vi "Motor Controller Mech Config.vi"(0 "COM port":refnum<visa-resource-name>, 5 "RS-485 addr.":u8, 7 "Encoder counting edges":u8=4, 9 "Encoder PPR":u16=256, 11 "Final drive ratio (X:1)":sgl=1.0, 12 "Close port after action":bool) -> (4 "COM port out":refnum<visa-resource-name>, 15 "Error out":errorcluster)   [LabVIEW 2020]
uses:
  ctls/CTRL_Cmd.ctl
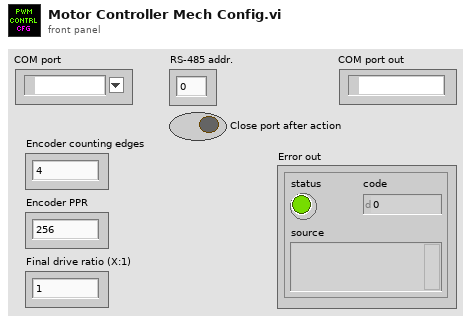
[diagram p1: front panel]
types:
  T1 = typedef "CTRL_Cmd.ctl" = string
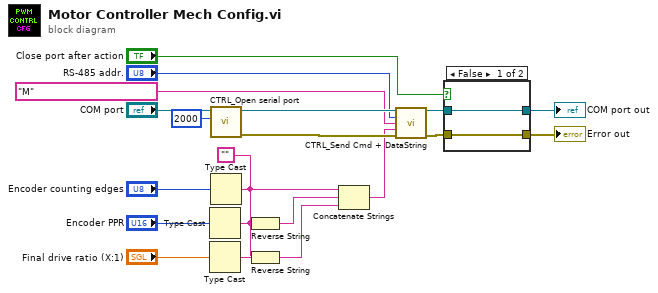
[diagram p0: block diagram]
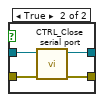
[diagram p2: hidden frame]
diagram:
  w8 = ""
  n1 = Type Cast(type=w8, x="Encoder PPR") -> (*(type *) &x=w14:string)
  n2 = Type Cast(type=w8, x="Final drive ratio (X:1)") -> (*(type *) &x=w13:string)
  n3 = call "CTRL_Open serial port.vi"("timeout (ms)"=u32 2000, "VISA resource name"="COM port") -> ("Error out"=w18:errorcluster, "VISA resource name out"=w19:refnum<visa-resource-name>)  [unwired: 8 in]
  n4 = Type Cast(type=w8, x="Encoder counting edges") -> (*(type *) &x=w9:string)
  n5 = Reverse String(1:w14) -> (0:w12:string)
  n6 = Reverse String(1:w13) -> (0:w11:string)
  n7 = Concatenate Strings(w9, w12, w11) -> (w10:string)
  n8 = call "CTRL_Send Cmd + DataString.vi"("Port"=w19, "RS-485 addr."="RS-485 addr.", "Cmd"=T1 "M", "DataString"=w10, "Error In"=w18) -> ("Port out"=w16:refnum<visa-resource-name>, "Error Out"=w15:errorcluster)  [unwired: 9 in]
  n9 = case shown="False" "Close port after action" {
    tunnel: [w23 w26] -> w17
    tunnel: w16 -> [w22 w24]
    tunnel: w15 -> [w23 w25]
    tunnel: [w22 w24] -> w1
    frame False {
    }
    frame True {
      n10 = call "CTRL_Close serial port.vi"("Error in"=w25, "VISA resource name"=w24) -> ("Error out"=w26:errorcluster)  [unwired: 9 in]
    }
  }
  "Error out" <- w17
  "COM port out" <- w1
